vi "ON_OFF_Trigger_toPVCAM.vi"(11 "Trigger":T1) -> (3 "trigger mode (input)":T2)   [LabVIEW 2013, in "Photometrics_CH-250_Cam.lvclass"]
doc: "Convert the \"ON/OFF\" trigger to a PVCAM compatible trigger"
uses:
  Photometrics_CH-250_Cam.lvclass
  TriggerMode_TypDef.ctl
  shared/OnOffTypeDef.ctl
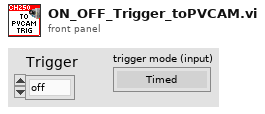
[diagram p1: front panel]
types:
  T1 = typedef "OnOffTypeDef.ctl" = enum16{"off", "on"}
  T2 = typedef "TriggerMode_TypDef.ctl" = enum16{"Timed", "Strobed", "Bulb", "Trigger first", "Flash", "Variable Timed"}
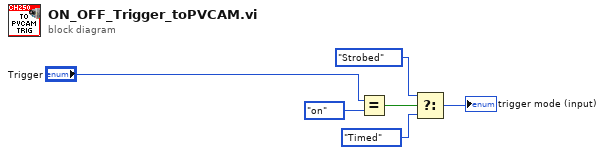
[diagram p0: block diagram]
diagram:
  n1 = Equal?(x="Trigger", y=OnOffTypeDef."on") -> (x = y?=w3:bool)
  n2 = Select(t=TriggerMode_TypDef."Strobed" ("trigger mode (input)"), s=w3, f=TriggerMode_TypDef."Timed" ("trigger mode (input)")) -> (s? t:f=→"trigger mode (input)":T2)
